vi "Configure Measurement (Occupied Bandwidth).vi"(0 "VISA resource name":refnum<visa-resource-name>, 1 "Max Hold (OFF)":bool, 5 "Occupied Bandwidth Percent Power (99%)":dbl=99.0 format="%#.6g", 7 "Occupied Bandwidth Span (3 MHz)":dbl=3000000.0 format="%#.6g", 9 "X dB (-26 dB)":dbl=-26.0 format="%#.6g", 11 "error in (no error)":errorcluster) -> (4 "VISA resource name out":refnum<visa-resource-name>, 15 "error out":errorcluster)   [LabVIEW 2014, in "Agilent ESA PSA Series.lvlib"]
doc: "Sets up the occupied bandwidth measurement operation."
uses:
  Agilent ESA PSA Series.lvlib
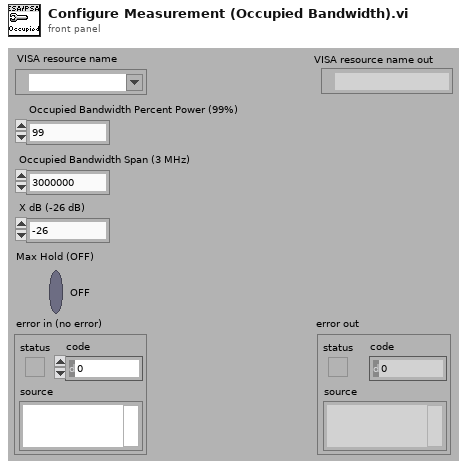
[diagram p1: front panel]
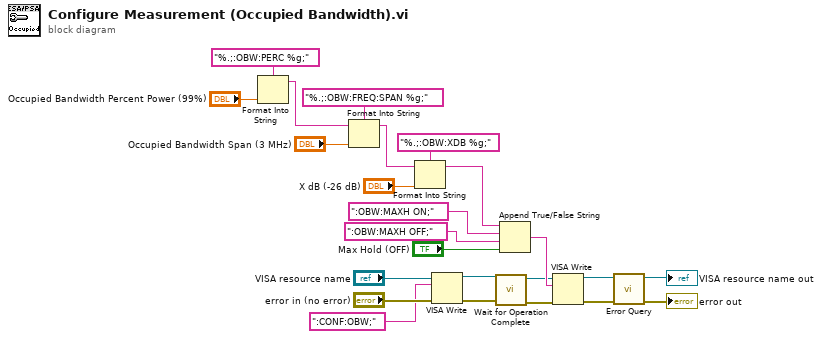
[diagram p0: block diagram]
diagram:
  n1 = Format Into String(format string="%.;:OBW:PERC %g;", "Occupied Bandwidth Percent Power (99%)") -> (resulting string=w20:string)  [unwired: 2 in, 1 out]
  n2 = Format Into String(format string="%.;:OBW:FREQ:SPAN %g;", initial string=w20, "Occupied Bandwidth Span (3 MHz)") -> (resulting string=w17:string)  [unwired: 1 in, 1 out]
  n3 = Format Into String(format string="%.;:OBW:XDB %g;", initial string=w17, "X dB (-26 dB)") -> (resulting string=w13:string)  [unwired: 1 in, 1 out]
  n4 = VISA Write(VISA resource name="VISA resource name", write buffer=":CONF:OBW;" ("initial string"), error in (no error)="error in (no error)") -> (VISA resource name out=w6:refnum<visa-resource-name>, error out=w7:errorcluster)  [unwired: 1 out]
  n5 = call "Wait for Operation Complete.vi"("error in (no error)"=w7, "VISA resource name"=w6) -> ("error out"=w4:errorcluster, "VISA resource name out"=w5:refnum<visa-resource-name>)  [unwired: 8 in]
  n6 = Append True/False String(1:"Max Hold (OFF)", 2:":OBW:MAXH OFF;", 3:":OBW:MAXH ON;", 4:w13) -> (0:w10:string)
  n7 = VISA Write(VISA resource name=w5, write buffer=w10, error in (no error)=w4) -> (VISA resource name out=w9:refnum<visa-resource-name>, error out=w8:errorcluster)  [unwired: 1 out]
  n8 = call "Error Query.vi"("error in (no error)"=w8, "VISA resource name"=w9) -> ("error out"=→"error out":errorcluster, "VISA resource name out"=→"VISA resource name out":refnum<visa-resource-name>)  [unwired: 6 in, 2 out]
